vi "Drive Brake.vi"(1 "Butterfly_State_In":bool) -> (0 "Butterfly_State_Out":bool)   [LabVIEW 2018]
uses:
  RefNumsDriverStation.vi
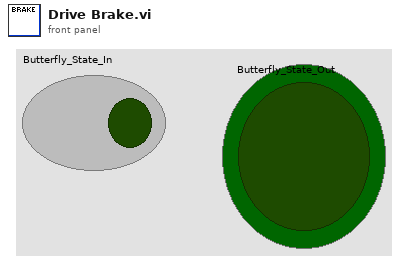
[diagram p1: front panel]
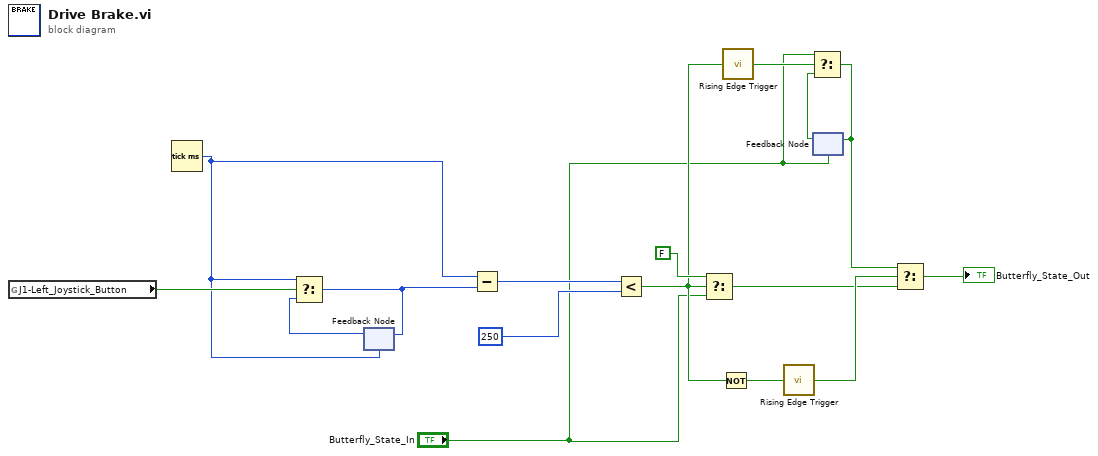
[diagram p0: block diagram]
diagram:
  n1 = global read "RefNumsDriverStation.vi" "J1-Left_Joystick_Button"() -> (w15:bool)
  n2 = Tick Count (ms)() -> (millisecond timer value=w14:u32)
  n3 = feedback #1(w14) -> (w16:u32)
  n4 = Select(t=w14, s=w15, f=w16) -> (s? t:f=w13:u32)
  n5 = feedback-in #1(w13) -> ()
  n6 = Subtract(x=w14, y=w13) -> (x-y=w12:u32)
  n7 = Less?(x=w12, y=u32 250) -> (x < y?=w6:bool)
  n8 = Select(t=FALSE, s=w6, f="Butterfly_State_In") -> (s? t:f=w7:bool)
  n9 = Not(x=w6) -> (.not. x?=w9:bool)
  n10 = call "Rising Edge Trigger.vi"("Raw Signal"=w6) -> ("Trigger"=w5:bool)
  n11 = call "Rising Edge Trigger.vi"("Raw Signal"=w9) -> ("Trigger"=w8:bool)
  n12 = feedback #2("Butterfly_State_In") -> (w4:bool)
  n13 = Select(t="Butterfly_State_In", s=w5, f=w4) -> (s? t:f=w3:bool)
  n14 = feedback-in #2(w3) -> ()
  n15 = Select(t=w3, s=w8, f=w7) -> (s? t:f=→"Butterfly_State_Out":bool)
